vi "route.vi"() -> ()   [LabVIEW 2014]
uses:
  <vilib>/Utility/sysdir.llb/System Directory Type.ctl
  <vilib>/Utility/config.llb/Read Key (Path).vi
  subVI/departure.vi
  subVI/Destination.vi
  <vilib>/Utility/file.llb/Write To Spreadsheet File (string).vi
  <vilib>/Utility/config.llb/Write Key (Path).vi
  <vilib>/httpClient/LabVIEWHTTPClient.lvlib
  <vilib>/Utility/config.llb/NI_LVConfig.lvlib
panel:
  out "fms":string
  in  "날시":bool
  out "FUEL/연료":i32
  out "time/시간":dbl
  in  "도움말":bool
  in  "피드백":bool
  in  "저장 경로":path
  out "Distance":string="0"
  in  "찾기":bool
  in  "?":bool
  in  "?":bool
  out "x fmc 플랜":string
  out "FMS 플랜":string
  in  "Destination":string
  in  "departure":string
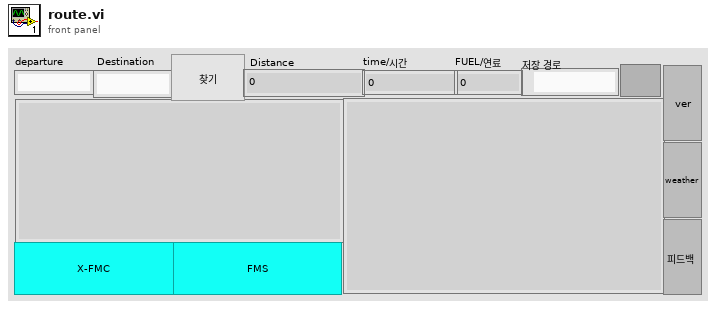
[diagram p1: front panel]
types:
  T1 = enum16{"open", "replace", "create", "open or create", "replace or create", "replace or create with confirmation"}
  T2 = typedef "System Directory Type.ctl" = i32
  T3 = typedef "NI_LVConfig.lvlib/Config Data RefNum.ctl" = refnum<k1>
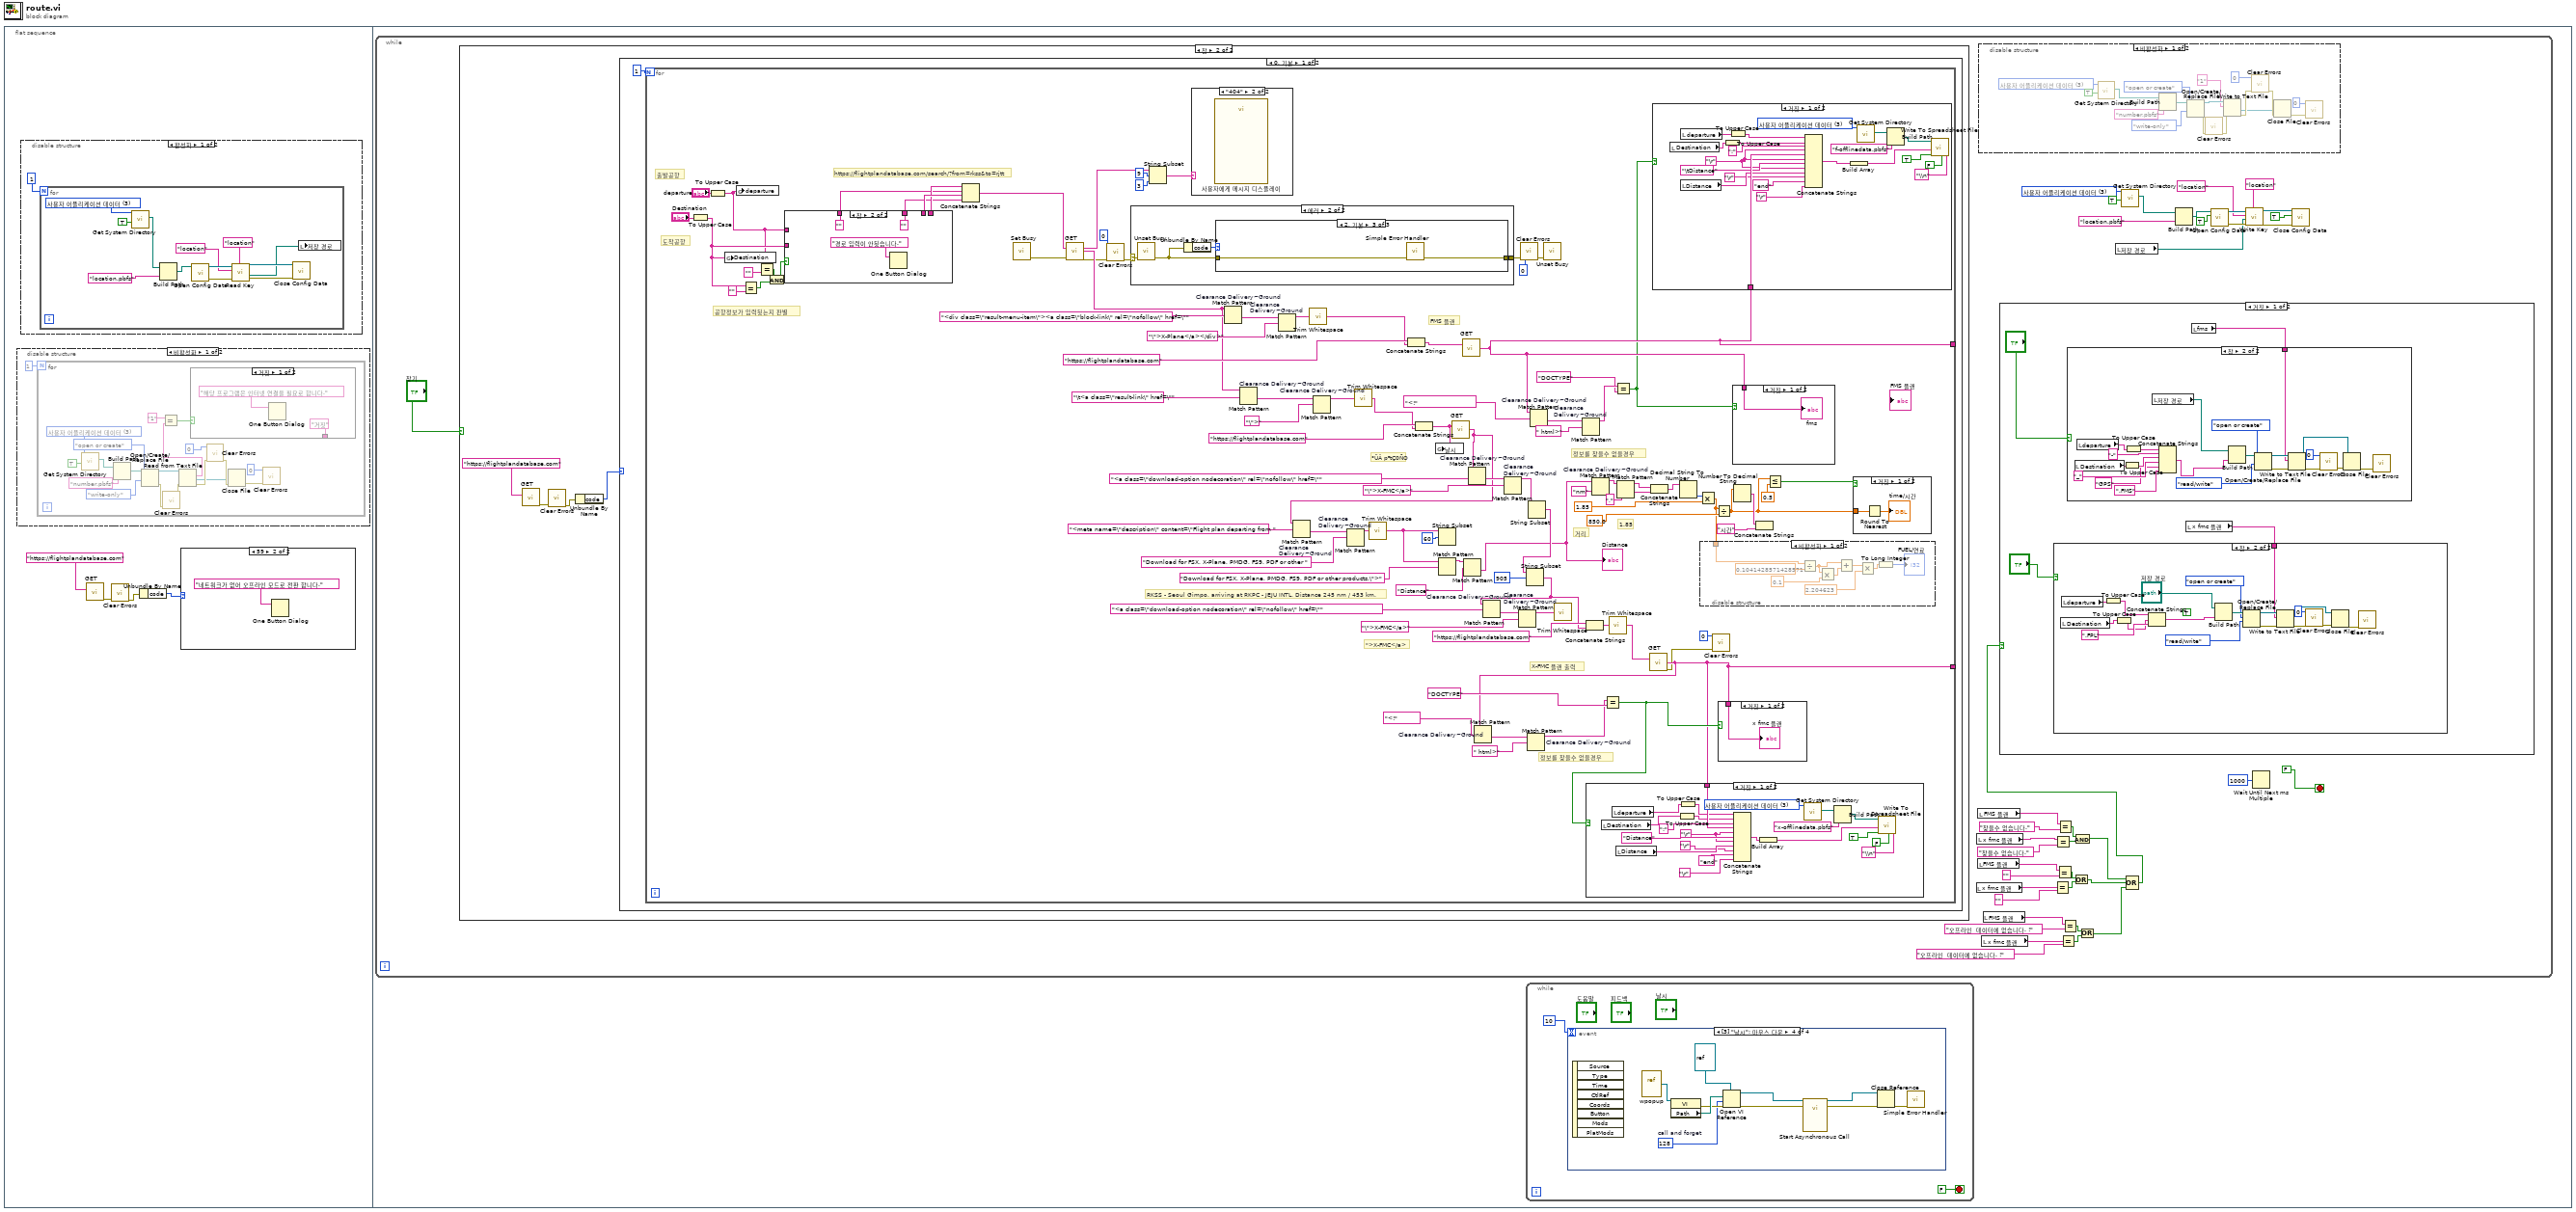
[diagram p0: block diagram]
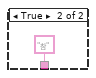
[diagram p3: hidden frame]
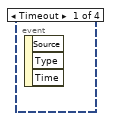
[diagram p6: hidden frame]
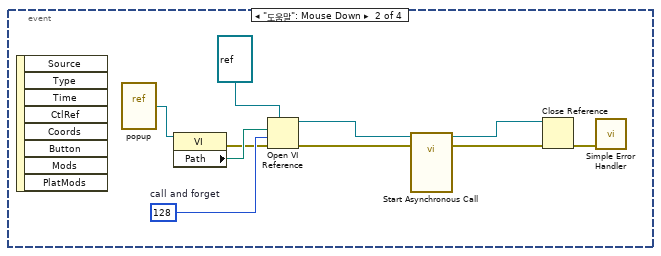
[diagram p7: hidden frame]
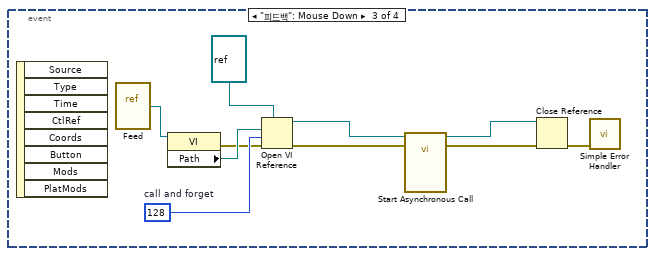
[diagram p8: hidden frame]
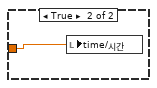
[diagram p13: hidden frame]
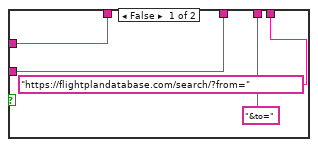
[diagram p14: hidden frame]
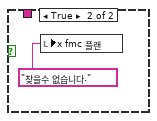
[diagram p15: hidden frame]
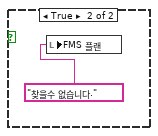
[diagram p16: hidden frame]
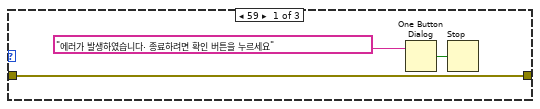
[diagram p19: hidden frame]
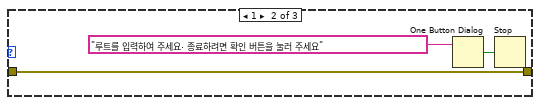
[diagram p20: hidden frame]
diagram:
  n1 = flat-sequence {
    frame #0 {
      n2 = disable-structure shown="비활성화" {
        frame Disabled {
          n3 = for {
            N: 1 -> [_]
            w12 = T2 3 items=["사용자 홈"=0, "사용자 데스크탑"=1, "사용자 문서"=2, "사용자 어플리케이션 데이터"=3, "사용자 환경"=4, "사용자 임시"=5, "퍼블릭 문서"=6, "퍼블릭 어플리케이션 데이터"=7, "퍼블릭 환경"=8, "퍼블릭 캐시"=13, "시스템 코어 라이브러리"=9, "시스템 설치된 라이브러리"=10, "어플리케이션 파일"=11, "부팅 볼륨 루트"=12] ("system directory type")
            n4 = call <vilib>:"Get System Directory.vi"("create directory if not found? (F)"=TRUE, "system directory type"=w12) -> ("system directory"=w13:path)  [unwired: 9 in]
            n5 = Build Path(base path=w13, name or relative path="number.pbfs" ("이름 또는 상대 경로")) -> (appended path=w18:path)
            n6 = Open/Create/Replace File(file path (use dialog)=w18, operation (0:open)=T1."open or create" ("동작(0:open)"), access (0:read/write)=enum16{"read/write", "read-only", "write-only"}."write-only" ("접근(0:읽기/쓰기)")) -> (refnum out=w21:refnum<file>, error out=w10:errorcluster)  [unwired: 3 in, 1 out]
            n7 = call <vilib>:"Clear Errors.vi"("error in (no error)"=w10) -> ("error out"=w9:errorcluster)  [unwired: 5 in, 1 out]
            n8 = Read from Text File(file (use dialog)=w21, error in=w9) -> (refnum out=w22:refnum<file>, text=w7:string, error out=w23:errorcluster)  [unwired: 2 in, 1 out]
            n9 = Equal?(x="1" ("y"), y=w7) -> (x = y?=w17:bool)
            n10 = case shown="거짓" w17 {
              tunnel: ["거짓" "참"] -> _
              frame False {
                n11 = One Button Dialog(message="해당 프로그램은 인터넷 연결을 필요로 합니다." ("메시지")) -> ()  [unwired: 1 in, 1 out]
              }
              frame True {
              }
            }
            n12 = call <vilib>:"Clear Errors.vi"("error in (no error)"=w23, "specific error code to clear (0: all)"=0) -> ("error out"=w24:errorcluster)  [unwired: 4 in, 1 out]
            n13 = Close File(refnum=w22, error in=w24) -> (error out=w15:errorcluster)  [unwired: 1 out]
            n14 = call <vilib>:"Clear Errors.vi"("error in (no error)"=w15, "specific error code to clear (0: all)"=0) -> ()  [unwired: 4 in, 2 out]
          }
        }
        frame Enabled {
        }
      }
      n15 = disable-structure shown="활성화" {
        frame Enabled {
          n16 = for {
            N: 1 -> [_]
            w40 = T2 3 items=["사용자 홈"=0, "사용자 데스크탑"=1, "사용자 문서"=2, "사용자 어플리케이션 데이터"=3, "사용자 환경"=4, "사용자 임시"=5, "퍼블릭 문서"=6, "퍼블릭 어플리케이션 데이터"=7, "퍼블릭 환경"=8, "퍼블릭 캐시"=13, "시스템 코어 라이브러리"=9, "시스템 설치된 라이브러리"=10, "어플리케이션 파일"=11, "부팅 볼륨 루트"=12] ("system directory type")
            n17 = call <vilib>:"Get System Directory.vi"("create directory if not found? (F)"=TRUE, "system directory type"=w40) -> ("system directory"=w38:path)  [unwired: 9 in]
            n18 = Build Path(base path=w38, name or relative path="location.pbfs" ("문자열")) -> (appended path=w37:path)
            n19 = call <vilib>:"Open Config Data.vi"("configuration file path"=w37) -> ("error out"=w34:errorcluster, "refnum"=w33:T3)  [unwired: 8 in, 1 out]
            n20 = call-poly <vilib>:"Read Key.vi"("section"="location", "error in (no error)"=w34, "key"="location", "refnum"=w33) -> ("error out"=w35:errorcluster, "value"=w30:path, "refnum out"=w36:T3)  [unwired: 4 in, 1 out]
            n21 = call <vilib>:"Close Config Data.vi"("error in (no error)"=w35, "refnum"=w36) -> ()  [unwired: 8 in, 2 out]
            n22 = local write "저장 경로"(w30) -> ()
          }
        }
        frame Disabled {
        }
      }
      n23 = call <vilib>:"GET.vi"("url"="https://flightplandatabase.com") -> ("error out"=w4:errorcluster)  [unwired: 11 in, 3 out]
      n24 = call <vilib>:"Clear Errors.vi"("error in (no error)"=w4) -> ("error out"=w2:errorcluster)  [unwired: 5 in, 1 out]
      n25 = Unbundle By Name(w2) -> ("code"=w1:i32)
      n26 = case shown="59" w1 {
        frame 0, Default {
        }
        frame 59 {
          n27 = One Button Dialog(message="네트워크가 없어 오프라인 모드로 전환 합니다." ("메시지")) -> ()  [unwired: 1 in, 1 out]
        }
      }
    }
    frame #1 {
      n28 = while {
        stop <- FALSE stop-if-true
        w94 = T2 3 items=["사용자 홈"=0, "사용자 데스크탑"=1, "사용자 문서"=2, "사용자 어플리케이션 데이터"=3, "사용자 환경"=4, "사용자 임시"=5, "퍼블릭 문서"=6, "퍼블릭 어플리케이션 데이터"=7, "퍼블릭 환경"=8, "퍼블릭 캐시"=13, "시스템 코어 라이브러리"=9, "시스템 설치된 라이브러리"=10, "어플리케이션 파일"=11, "부팅 볼륨 루트"=12] ("system directory type")
        n29 = case shown="참" "찾기" {
          frame False {
          }
          frame True {
            n30 = call <vilib>:"GET.vi"("url"="https://flightplandatabase.com") -> ("error out"=w116:errorcluster)  [unwired: 11 in, 3 out]
            n31 = call <vilib>:"Clear Errors.vi"("error in (no error)"=w116) -> ("error out"=w114:errorcluster)  [unwired: 5 in, 1 out]
            n32 = Unbundle By Name(w114) -> ("code"=w113:i32)
            n33 = case shown="0, 기본" w113 {
              frame 0, Default {
                n34 = for {
                  N: 1 -> [_]
                  tunnel: [w126] -> _
                  tunnel: [w132] -> _
                  # "°ÜÂ p³tÇ0ÑO"
                  # "1.85"
                  # "RKSS - Seoul Gimpo, arriving at RKPC - JEJU INTL. Distance 245 nm / 453 km."
                  # "\">X-FMC</a>"
                  # "https://flightplandatabase.com/search/?from=rkss&to=rjtt"
                  # "FMS 플랜"
                  # "거리"
                  # "X-FMC 플랜 출력"
                  # "정보를 찾을수 없을경우"
                  # "정보를 찾을수 없을경우"
                  # "공항정보가 입력됫는지 판별"
                  # "도착공항"
                  # "출발공항"
                  n35 = To Upper Case(1:"Destination") -> (0:w120:string)
                  n36 = To Upper Case(1:"departure") -> (0:w119:string)
                  n37 = global write "Destination.vi" "Destination"(w120) -> ()
                  n38 = global write "departure.vi" "departure"(w119) -> ()
                  n39 = Equal?(x=w120, y="") -> (x = y?=w158:bool)
                  n40 = Equal?(x=w119, y="") -> (x = y?=w157:bool)
                  n41 = And(x=w157, y=w158) -> (x .and. y?=w159:bool)
                  n42 = case shown="참" w159 {
                    tunnel: ["&to=" ("문자열") _] -> w149
                    tunnel: ["https://flightplandatabase.com/search/?from=" ("문자열") _] -> w148
                    tunnel: w120 -> [w269 _]
                    tunnel: [w269 "" ("Destination")] -> w147
                    tunnel: [w268 "" ("departure")] -> w146
                    tunnel: w119 -> [w268 _]
                    frame False {
                    }
                    frame True {
                      n43 = One Button Dialog(message="경로 입력이 안됫습니다." ("메시지")) -> ()  [unwired: 1 in, 1 out]
                    }
                  }
                  n44 = Concatenate Strings(w148, w146, w149, w147) -> (w130:string)
                  n45 = call <vilib>:"Set Busy.vi"() -> ("error out"=w209:errorcluster)  [unwired: 10 in, 1 out]
                  n46 = call <vilib>:"GET.vi"("url"=w130, "error in (no error)"=w209) -> ("headers"=w213:string, "body"=w183:string, "error out"=w168:errorcluster)  [unwired: 10 in, 1 out]
                  n47 = call <vilib>:"Clear Errors.vi"("error in (no error)"=w168, "specific error code to clear (0: all)"=0) -> ("error out"=w169:errorcluster)  [unwired: 4 in, 1 out]
                  n48 = case shown="에러" w169 {
                    selector: w169 -> [w279 w282]
                    tunnel: [w279 w280] -> w165
                    frame No Error {
                    }
                    frame Error {
                      n49 = call <vilib>:"Unset Busy.vi"("error in (no error)"=w282) -> ("error out"=w281:errorcluster)  [unwired: 10 in]
                      n50 = Unbundle By Name(w281) -> ("code"=w283:i32)
                      n51 = case shown="2, 기본" w283 {
                        tunnel: w281 -> [w284 w289 w291]
                        tunnel: [w284 w289 w290] -> w280
                        frame 59 {
                          n52 = One Button Dialog(message="에러가 발생하였습니다. 종료하려면 확인 버튼을 누르세요" ("메시지")) -> (true=w285:bool)  [unwired: 1 in]
                          n53 = Stop(stop? (T)=w285) -> ()
                        }
                        frame 1 {
                          n54 = One Button Dialog(message="루트를 입력하여 주세요. 종료하려면 확인 버튼을 눌러 주세요" ("메시지")) -> (true=w287:bool)  [unwired: 1 in]
                          n55 = Stop(stop? (T)=w287) -> ()
                        }
                        frame 2, Default {
                          n56 = call <vilib>:"Simple Error Handler.vi"("error in (no error)"=w291) -> ("error out"=w290:errorcluster)  [unwired: 4 in, 4 out]
                        }
                      }
                    }
                  }
                  n57 = String Subset(string=w213, offset (0)=9 ("오프셋(0)"), length (rest)=3 ("길이(나머지)")) -> (substring=w210:string)
                  n58 = case shown="\"404\"" w210 {
                    frame "거짓", Default {
                    }
                    frame "404" {
                      n59 = call "사용자에게 메시지 디스플레이"() -> ()  [unwired: 10 in, 2 out]
                    }
                  }
                  n60 = Match Pattern "Clearance Delivery~Ground"(string=w183, regular expression="<div class=\"result-menu-item\"><a class=\"block-link\" rel=\"nofollow\" href=\"" ("정규식")) -> (after substring=w207:string)  [unwired: 1 in, 3 out]
                  n61 = Match Pattern "Clearance Delivery~Ground"(string=w183, regular expression="\t<a class=\"result-link\" href=\"" ("정규식")) -> (after substring=w201:string)  [unwired: 1 in, 3 out]
                  n62 = Match Pattern "Clearance Delivery~Ground"(string=w207, regular expression="\">X-Plane</a></div>" ("정규식")) -> (before substring=w205:string)  [unwired: 1 in, 3 out]
                  n63 = call <vilib>:"Trim Whitespace.vi"("string"=w205) -> ("trimmed string"=w202:string)  [unwired: 1 in]
                  n64 = Match Pattern "Clearance Delivery~Ground"(string=w201, regular expression="\">" ("정규식")) -> (before substring=w198:string)  [unwired: 1 in, 3 out]
                  n65 = call <vilib>:"Trim Whitespace.vi"("string"=w198) -> ("trimmed string"=w196:string)  [unwired: 1 in]
                  n66 = Concatenate Strings("https://flightplandatabase.com" ("url"), w202) -> (w203:string)
                  n67 = Concatenate Strings("https://flightplandatabase.com" ("url"), w196) -> (w128:string)
                  n68 = global write "날시.vi" "날시"(w128) -> ()
                  n69 = call <vilib>:"GET.vi"("url"=w128) -> ("body"=w129:string)  [unwired: 11 in, 3 out]
                  n70 = Match Pattern "Clearance Delivery~Ground"(string=w129, regular expression="<meta name=\"description\" content=\"Flight plan departing from " ("정규식")) -> (after substring=w184:string)  [unwired: 1 in, 3 out]
                  n71 = Match Pattern "Clearance Delivery~Ground"(string=w184, regular expression="Download for FSX, X-Plane, PMDG, FS9, PDF or other " ("정규식")) -> (before substring=w186:string)  [unwired: 1 in, 3 out]
                  n72 = call <vilib>:"Trim Whitespace.vi"("string"=w186) -> ("trimmed string"=w154:string)  [unwired: 1 in]
                  n73 = String Subset(string=w154, offset (0)=60 ("오프셋(0)")) -> ()  [unwired: 1 in, 1 out]
                  n74 = Match Pattern(string=w154, regular expression="Download for FSX, X-Plane, PMDG, FS9, PDF or other products.\">" ("정규식")) -> (before substring=w152:string)  [unwired: 1 in, 3 out]
                  n75 = call <vilib>:"GET.vi"("url"=w203) -> ("body"=w132:string)  [unwired: 11 in, 3 out]
                  n76 = Match Pattern(string=w152, regular expression="Distance" ("정규식")) -> (after substring=w150:string)  [unwired: 1 in, 3 out]
                  "Distance" <- w150
                  n77 = Match Pattern "Clearance Delivery~Ground"(string=w129, regular expression="<a class=\"download-option nodecoration\" rel=\"nofollow\" href=\"" ("정규식")) -> (after substring=w193:string)  [unwired: 1 in, 3 out]
                  n78 = Match Pattern "Clearance Delivery~Ground"(string=w193, regular expression="\">X-FMC</a>" ("정규식")) -> (before substring=w192:string)  [unwired: 1 in, 3 out]
                  n79 = call <vilib>:"Clear Errors.vi"("error in (no error)"=w165, "specific error code to clear (0: all)"=0) -> ("error out"=w166:errorcluster)  [unwired: 4 in, 1 out]
                  n80 = String Subset(string=w192) -> (substring=w155:string)  [unwired: 2 in]
                  n81 = String Subset(string=w155, offset (0)=905 ("오프셋(0)")) -> (substring=w122:string)  [unwired: 1 in]
                  n82 = Match Pattern "Clearance Delivery~Ground"(string=w122, regular expression="<a class=\"download-option nodecoration\" rel=\"nofollow\" href=\"" ("정규식")) -> (after substring=w189:string)  [unwired: 1 in, 3 out]
                  n83 = Match Pattern "Clearance Delivery~Ground"(string=w189, regular expression="\">X-FMC</a>" ("정규식")) -> (before substring=w123:string)  [unwired: 1 in, 3 out]
                  n84 = Match Pattern "Clearance Delivery~Ground"(string=w132, regular expression="<!" ("문자열")) -> (after substring=w179:string)  [unwired: 1 in, 3 out]
                  n85 = call <vilib>:"Unset Busy.vi"("error in (no error)"=w166) -> ()  [unwired: 10 in, 1 out]
                  n86 = call <vilib>:"Trim Whitespace.vi"("string"=w123) -> ()  [unwired: 1 in, 1 out]
                  n87 = Match Pattern "Clearance Delivery~Ground"(string=w179, regular expression=" html>" ("정규식")) -> (before substring=w178:string)  [unwired: 1 in, 3 out]
                  n88 = Concatenate Strings("https://flightplandatabase.com" ("url"), w122) -> (w187:string)
                  n89 = Match Pattern "Clearance Delivery~Ground"(string=w150, regular expression="nm" ("정규식")) -> (before substring=w142:string)  [unwired: 1 in, 3 out]
                  n90 = call <vilib>:"Trim Whitespace.vi"("string"=w187) -> ("trimmed string"=w127:string)  [unwired: 1 in]
                  n91 = Equal?(x=w178, y="DOCTYPE") -> (x = y?=w131:bool)
                  n92 = Match Pattern(string=w142, regular expression="," ("정규식")) -> (before substring=w139:string, after substring=w138:string)  [unwired: 1 in, 2 out]
                  n93 = call <vilib>:"GET.vi"("url"=w127) -> ("body"=w126:string, "error out"=w125:errorcluster)  [unwired: 11 in, 2 out]
                  n94 = Match Pattern "Clearance Delivery~Ground"(string=w126, regular expression="<!" ("문자열")) -> (after substring=w176:string)  [unwired: 1 in, 3 out]
                  n95 = Match Pattern "Clearance Delivery~Ground"(string=w176, regular expression=" html>" ("정규식")) -> (before substring=w173:string)  [unwired: 1 in, 3 out]
                  n96 = Equal?(x=w173, y="DOCTYPE") -> (x = y?=w133:bool)
                  n97 = case shown="거짓" w133 {
                    tunnel: w126 -> [w254 _]
                    frame False {
                      w248 = "\r"
                      w257 = T2 3 items=["사용자 홈"=0, "사용자 데스크탑"=1, "사용자 문서"=2, "사용자 어플리케이션 데이터"=3, "사용자 환경"=4, "사용자 임시"=5, "퍼블릭 문서"=6, "퍼블릭 어플리케이션 데이터"=7, "퍼블릭 환경"=8, "퍼블릭 캐시"=13, "시스템 코어 라이브러리"=9, "시스템 설치된 라이브러리"=10, "어플리케이션 파일"=11, "부팅 볼륨 루트"=12] ("system directory type")
                      n98 = local read "Destination"() -> (w250:string)
                      n99 = local read "departure"() -> (w253:string)
                      n100 = local read "Distance"() -> (w247:string)
                      n101 = To Upper Case(1:w250) -> (0:w251:string)
                      n102 = To Upper Case(1:w253) -> (0:w252:string)
                      n103 = Concatenate Strings(w252, w251, ":", w254, w248, "Distance" ("문자열"), w248, w247, "\r", "end", "\r") -> (w255:string)
                      n104 = Build Array(w255) -> (w259:string[])
                      n105 = call <vilib>:"Get System Directory.vi"("system directory type"=w257) -> ("system directory"=w261:path)  [unwired: 10 in]
                      n106 = Build Path(base path=w261, name or relative path="x-offlinedata.pbfs" ("이름 또는 상대 경로")) -> (appended path=w260:path)
                      n107 = call-poly <vilib>:"Write To Spreadsheet File.vi"("delimiter (\\t)"="\\n" ("delimiter (\\t)"), "transpose? (no:F)"=FALSE, "append to file? (new file:F)"=TRUE, "1D data"=w259, "file path (dialog if empty)"=w260) -> ()  [unwired: 3 in, 1 out]
                    }
                    frame True {
                    }
                  }
                  n108 = Concatenate Strings(w139, w138) -> (w141:string)
                  n109 = case shown="거짓" w131 {
                    tunnel: w132 -> [w229 _]
                    frame False {
                      w227 = "\r"
                      w236 = T2 3 items=["사용자 홈"=0, "사용자 데스크탑"=1, "사용자 문서"=2, "사용자 어플리케이션 데이터"=3, "사용자 환경"=4, "사용자 임시"=5, "퍼블릭 문서"=6, "퍼블릭 어플리케이션 데이터"=7, "퍼블릭 환경"=8, "퍼블릭 캐시"=13, "시스템 코어 라이브러리"=9, "시스템 설치된 라이브러리"=10, "어플리케이션 파일"=11, "부팅 볼륨 루트"=12] ("system directory type")
                      n110 = local read "Destination"() -> (w230:string)
                      n111 = local read "Distance"() -> (w226:string)
                      n112 = local read "departure"() -> (w232:string)
                      n113 = To Upper Case(1:w230) -> (0:w231:string)
                      n114 = To Upper Case(1:w232) -> (0:w233:string)
                      n115 = Concatenate Strings(w233, w231, ":", w227, w229, w227, "\tDistance", w227, w226, "\r", "end", "\r") -> (w234:string)
                      n116 = Build Array(w234) -> (w238:string[])
                      n117 = call <vilib>:"Get System Directory.vi"("system directory type"=w236) -> ("system directory"=w240:path)  [unwired: 10 in]
                      n118 = Build Path(base path=w240, name or relative path="f-offlinedata.pbfs" ("이름 또는 상대 경로")) -> (appended path=w239:path)
                      n119 = call-poly <vilib>:"Write To Spreadsheet File.vi"("delimiter (\\t)"="\\n" ("delimiter (\\t)"), "transpose? (no:F)"=FALSE, "append to file? (new file:F)"=TRUE, "1D data"=w238, "file path (dialog if empty)"=w239) -> ()  [unwired: 3 in, 1 out]
                    }
                    frame True {
                    }
                  }
                  n120 = Decimal String To Number(string=w141) -> (number=w143:i32)  [unwired: 2 in, 1 out]
                  n121 = Multiply(x=w143, y=1.85) -> (x*y=w134:dbl)
                  n122 = disable-structure shown="비활성화" {
                    disable-tunnel: w134 -> [w219 _]
                    frame Disabled {
                      n123 = Divide(x=w219, y=0.1041428571428571) -> (x/y=w220:dbl)
                      n124 = Multiply(x=w220, y=0.1) -> (x*y=w218:dbl)
                      n125 = Add(x=w220, y=w218) -> (x+y=w217:dbl)
                      n126 = Multiply(x=w217, y=2.204623) -> (x*y=w214:dbl)
                      n127 = To Long Integer(number=w214) -> (32bit integer=→"FUEL/연료":i32)
                    }
                    frame Enabled {
                    }
                  }
                  n128 = call <vilib>:"Clear Errors.vi"("error in (no error)"=w125, "specific error code to clear (0: all)"=0) -> ()  [unwired: 4 in, 2 out]
                  n129 = Divide(x=w134, y=850.0) -> (x/y=w135:dbl)
                  n130 = case shown="거짓" w133 {
                    tunnel: w126 -> [w275 _]
                    frame False {
                      "x fmc 플랜" <- w275
                    }
                    frame True {
                      n131 = local write "x fmc 플랜"("찾을수 없습니다.") -> ()
                    }
                  }
                  n132 = case shown="거짓" w131 {
                    tunnel: w132 -> [w277 _]
                    frame False {
                      "fms" <- w277
                    }
                    frame True {
                      n133 = local write "FMS 플랜"("찾을수 없습니다.") -> ()
                    }
                  }
                  n134 = Number To Decimal String(number=w135) -> (decimal integer string=w160:string)  [unwired: 1 in]
                  n135 = Concatenate Strings(w160, "시간") -> ()  [unwired: 1 out]
                  n136 = Less Or Equal?(x=w135, y=0.5) -> (x <= y?=w137:bool)
                  n137 = case shown="거짓" w137 {
                    tunnel: w135 -> [w266 w267]
                    frame False {
                      n138 = Round To Nearest(number=w266) -> (nearest integer value=→"time/시간":dbl)
                    }
                    frame True {
                      n139 = local write "time/시간"(w267) -> ()
                    }
                  }
                }
              }
              frame 59 {
                n140 = while {
                  stop <- FALSE stop-if-true
                  w292 = "Distance" ("정규식")
                  w329 = T2 1 items=["사용자 홈"=0, "사용자 데스크탑"=1, "사용자 문서"=2, "사용자 어플리케이션 데이터"=3, "사용자 환경"=4, "사용자 임시"=5, "퍼블릭 문서"=6, "퍼블릭 어플리케이션 데이터"=7, "퍼블릭 환경"=8, "퍼블릭 캐시"=13, "시스템 코어 라이브러리"=9, "시스템 설치된 라이브러리"=10, "어플리케이션 파일"=11, "부팅 볼륨 루트"=12] ("system directory type")
                  w343 = T2 1 items=["사용자 홈"=0, "사용자 데스크탑"=1, "사용자 문서"=2, "사용자 어플리케이션 데이터"=3, "사용자 환경"=4, "사용자 임시"=5, "퍼블릭 문서"=6, "퍼블릭 어플리케이션 데이터"=7, "퍼블릭 환경"=8, "퍼블릭 캐시"=13, "시스템 코어 라이브러리"=9, "시스템 설치된 라이브러리"=10, "어플리케이션 파일"=11, "부팅 볼륨 루트"=12] ("system directory type")
                  n141 = local read "Destination"() -> (w323:string)
                  n142 = local read "departure"() -> (w325:string)
                  n143 = call <vilib>:"Get System Directory.vi"("system directory type"=w329) -> ("system directory"=w328:path)  [unwired: 10 in]
                  n144 = call <vilib>:"Get System Directory.vi"("system directory type"=w343) -> ("system directory"=w344:path)  [unwired: 10 in]
                  n145 = To Upper Case(1:w323) -> (0:w322:string)
                  n146 = Build Path(base path=w328, name or relative path="f-offlinedata.pbfs" ("이름 또는 상대 경로")) -> (appended path=w331:path)
                  n147 = To Upper Case(1:w325) -> (0:w324:string)
                  n148 = Build Path(base path=w344, name or relative path="x-offlinedata.pbfs" ("이름 또는 상대 경로")) -> (appended path=w341:path)
                  n149 = Concatenate Strings(w324, w322, ":") -> (w319:string)
                  n150 = Read from Text File(file (use dialog)=w331) -> (refnum out=w332:refnum<file>, text=w317:string, error out=w333:errorcluster)  [unwired: 3 in, 1 out]
                  n151 = Read from Text File(file (use dialog)=w341) -> (refnum out=w340:refnum<file>, text=w293:string, error out=w339:errorcluster)  [unwired: 3 in, 1 out]
                  n152 = Close File(refnum=w332, error in=w333) -> ()  [unwired: 2 out]
                  n153 = Close File(refnum=w340, error in=w339) -> ()  [unwired: 2 out]
                  n154 = Match Pattern(string=w293, regular expression=w319) -> (after substring=w321:string)  [unwired: 1 in, 3 out]
                  n155 = Match Pattern(string=w317, regular expression=w319) -> (after substring=w326:string)  [unwired: 1 in, 3 out]
                  n156 = Match Pattern(string=w326, regular expression="Distance") -> (before substring=w327:string)  [unwired: 1 in, 3 out]
                  n157 = Match Pattern(string=w321, regular expression=w292) -> (before substring=w320:string)  [unwired: 1 in, 3 out]
                  n158 = Match Pattern(string=w293, regular expression=w292) -> (after substring=w316:string)  [unwired: 1 in, 3 out]
                  n159 = Match Pattern(string=w316, regular expression="end" ("정규식")) -> (before substring=w306:string)  [unwired: 1 in, 3 out]
                  n160 = Equal?(x=w320, y="") -> (x = y?=w338:bool)
                  n161 = call <vilib>:"Trim Whitespace.vi"("string"=w306) -> ("trimmed string"=w312:string)  [unwired: 1 in]
                  n162 = Match Pattern "time/fuel"(string=w312, regular expression="nm" ("정규식")) -> (before substring=w308:string)  [unwired: 1 in, 3 out]
                  n163 = Match Pattern(string=w308, regular expression="," ("정규식")) -> (before substring=w310:string, after substring=w311:string)  [unwired: 1 in, 2 out]
                  n164 = Concatenate Strings(w310, w311) -> (w309:string)
                  n165 = Decimal String To Number(string=w309) -> (number=w297:i32)  [unwired: 2 in, 1 out]
                  n166 = Multiply(x=w297, y=1.85) -> (x*y=w296:dbl)
                  n167 = Divide(x=w296, y=850.0) -> (x/y=w294:dbl)
                  n168 = Equal?(x=w327, y="") -> (x = y?=w335:bool)
                  n169 = case shown="거짓" w335 {
                    tunnel: w327 -> [w346 _]
                    frame False {
                      n170 = local write "FMS 플랜"(w346) -> ()
                    }
                    frame True {
                      n171 = local write "x fmc 플랜"("오프라인  데이터에 없습니다. !" ("메시지")) -> ()
                    }
                  }
                  n172 = Divide(x=w296, y=0.1041428571428571) -> (x/y=w300:dbl)
                  n173 = Multiply(x=w300, y=0.1) -> (x*y=w301:dbl)
                  n174 = Add(x=w300, y=w301) -> (x+y=w302:dbl)
                  n175 = Multiply(x=w302, y=2.204623) -> (x*y=w304:dbl)
                  n176 = To Long Integer(number=w304) -> (32bit integer=w295:i32)
                  n177 = case shown="거짓" w338 {
                    tunnel: w320 -> [w353 _]
                    tunnel: w295 -> [w348 _]
                    tunnel: w294 -> [w349 _]
                    tunnel: w294 -> [w350 _]
                    frame False {
                      n178 = Less Or Equal?(x=w350, y=0.5) -> (x <= y?=w352:bool)
                      n179 = local write "x fmc 플랜"(w353) -> ()
                      n180 = case shown="거짓" w352 {
                        tunnel: w349 -> [w354 w356]
                        frame False {
                          n181 = Round To Nearest(number=w354) -> (nearest integer value=w355:dbl)
                          n182 = local write "time/시간"(w355) -> ()
                        }
                        frame True {
                          n183 = local write "time/시간"(w356) -> ()
                        }
                      }
                      n184 = local write "FUEL/연료"(w348) -> ()
                    }
                    frame True {
                      n185 = local write "x fmc 플랜"("오프라인  데이터에 없습니다. !" ("메시지")) -> ()
                    }
                  }
                }
              }
            }
          }
        }
        n186 = local read "x fmc 플랜"() -> (w101:string)
        n187 = local read "x fmc 플랜"() -> (w109:string)
        n188 = local read "FMS 플랜"() -> (w96:string)
        n189 = local read "FMS 플랜"() -> (w107:string)
        n190 = disable-structure shown="비활성화" {
          frame Disabled {
            w361 = T2 3 items=["사용자 홈"=0, "사용자 데스크탑"=1, "사용자 문서"=2, "사용자 어플리케이션 데이터"=3, "사용자 환경"=4, "사용자 임시"=5, "퍼블릭 문서"=6, "퍼블릭 어플리케이션 데이터"=7, "퍼블릭 환경"=8, "퍼블릭 캐시"=13, "시스템 코어 라이브러리"=9, "시스템 설치된 라이브러리"=10, "어플리케이션 파일"=11, "부팅 볼륨 루트"=12] ("system directory type")
            n191 = call <vilib>:"Get System Directory.vi"("create directory if not found? (F)"=TRUE, "system directory type"=w361) -> ("system directory"=w362:path)  [unwired: 9 in]
            n192 = Build Path(base path=w362, name or relative path="number.pbfs" ("이름 또는 상대 경로")) -> (appended path=w367:path)
            n193 = Open/Create/Replace File(file path (use dialog)=w367, operation (0:open)=T1."open or create" ("동작(0:open)"), access (0:read/write)=enum16{"read/write", "read-only", "write-only"}."write-only" ("접근(0:읽기/쓰기)")) -> (refnum out=w370:refnum<file>, error out=w359:errorcluster)  [unwired: 3 in, 1 out]
            n194 = call <vilib>:"Clear Errors.vi"("error in (no error)"=w359) -> ("error out"=w358:errorcluster)  [unwired: 5 in, 1 out]
            n195 = Write to Text File(file (use dialog)=w370, text="1" ("텍스트"), error in=w358) -> (refnum out=w371:refnum<file>, error out=w372:errorcluster)  [unwired: 1 in, 1 out]
            n196 = call <vilib>:"Clear Errors.vi"("error in (no error)"=w372, "specific error code to clear (0: all)"=0) -> ("error out"=w373:errorcluster)  [unwired: 4 in, 1 out]
            n197 = Close File(refnum=w371, error in=w373) -> (error out=w364:errorcluster)  [unwired: 1 out]
            n198 = call <vilib>:"Clear Errors.vi"("error in (no error)"=w364, "specific error code to clear (0: all)"=0) -> ()  [unwired: 4 in, 2 out]
          }
          frame Enabled {
          }
        }
        n199 = local read "x fmc 플랜"() -> (w78:string)
        n200 = local read "FMS 플랜"() -> (w74:string)
        n201 = Equal?(x=w101, y="") -> (x = y?=w103:bool)
        n202 = Equal?(x=w109, y="찾을수 없습니다.") -> (x = y?=w110:bool)
        n203 = Equal?(x=w96, y="") -> (x = y?=w102:bool)
        n204 = Equal?(x=w107, y="찾을수 없습니다.") -> (x = y?=w111:bool)
        n205 = Equal?(x=w78, y="오프라인  데이터에 없습니다. !") -> (x = y?=w76:bool)
        n206 = Equal?(x=w74, y="오프라인  데이터에 없습니다. !") -> (x = y?=w77:bool)
        n207 = Or(x=w102, y=w103) -> (x .or. y?=w91:bool)
        n208 = And(x=w111, y=w110) -> (x .and. y?=w98:bool)
        n209 = Or(x=w77, y=w76) -> (x .or. y?=w75:bool)
        n210 = local read "저장 경로"() -> (w82:path)
        n211 = call <vilib>:"Get System Directory.vi"("create directory if not found? (F)"=TRUE, "system directory type"=w94) -> ("system directory"=w92:path)  [unwired: 9 in]
        n212 = Compound Arithmetic op=OR(w98, w91, w75) -> (w97:bool)
        n213 = case shown="거짓" w97 {
          frame False {
            n214 = local read "x fmc 플랜"() -> (w375:string)
            n215 = case shown="참" "?" {
              tunnel: w375 -> [_ w401]
              frame False {
              }
              frame True {
                (unwired) TRUE ("create directory if not found? (F)")
                n216 = local read "Destination"() -> (w408:string)
                n217 = local read "departure"() -> (w409:string)
                n218 = To Upper Case(1:w409) -> (0:w400:string)
                n219 = To Upper Case(1:w408) -> (0:w407:string)
                n220 = Concatenate Strings(w400, w407, ".FPL" ("문자열")) -> (w412:string)
                n221 = Build Path(base path="저장 경로", name or relative path=w412) -> (appended path=w415:path)
                n222 = Open/Create/Replace File(file path (use dialog)=w415, operation (0:open)=T1."open or create" ("동작(0:open)"), access (0:read/write)=enum16{"read/write", "read-only", "write-only"}."read/write" ("접근(0:읽기/쓰기)")) -> (refnum out=w417:refnum<file>, error out=w416:errorcluster)  [unwired: 3 in, 1 out]
                n223 = Write to Text File(file (use dialog)=w417, text=w401, error in=w416) -> (refnum out=w404:refnum<file>, error out=w406:errorcluster)  [unwired: 1 in, 1 out]
                n224 = call <vilib>:"Clear Errors.vi"("error in (no error)"=w406, "specific error code to clear (0: all)"=0) -> ("error out"=w405:errorcluster)  [unwired: 4 in, 1 out]
                n225 = Close File(refnum=w404, error in=w405) -> (error out=w402:errorcluster)  [unwired: 1 out]
                n226 = call <vilib>:"Clear Errors.vi"("error in (no error)"=w402) -> ()  [unwired: 5 in, 2 out]
              }
            }
            n227 = local read "fms"() -> (w377:string)
            n228 = case shown="참" "?" {
              tunnel: w377 -> [_ w394]
              frame False {
              }
              frame True {
                n229 = local read "Destination"() -> (w391:string)
                n230 = local read "departure"() -> (w390:string)
                n231 = To Upper Case(1:w391) -> (0:w382:string)
                n232 = To Upper Case(1:w390) -> (0:w384:string)
                n233 = local read "저장 경로"() -> (w386:path)
                n234 = Concatenate Strings(w384, "-" ("문자열"), w382, "_" ("문자열"), "GPS" ("문자열"), ".FMS" ("문자열")) -> (w392:string)
                n235 = Build Path(base path=w386, name or relative path=w392) -> (appended path=w396:path)
                n236 = Open/Create/Replace File(file path (use dialog)=w396, operation (0:open)=T1."open or create" ("동작(0:open)"), access (0:read/write)=enum16{"read/write", "read-only", "write-only"}."read/write" ("접근(0:읽기/쓰기)")) -> (refnum out=w399:refnum<file>, error out=w398:errorcluster)  [unwired: 3 in, 1 out]
                n237 = Write to Text File(file (use dialog)=w399, text=w394, error in=w398) -> (refnum out=w397:refnum<file>, error out=w389:errorcluster)  [unwired: 1 in, 1 out]
                n238 = call <vilib>:"Clear Errors.vi"("error in (no error)"=w389, "specific error code to clear (0: all)"=0) -> ("error out"=w388:errorcluster)  [unwired: 4 in, 1 out]
                n239 = Close File(refnum=w397, error in=w388) -> (error out=w385:errorcluster)  [unwired: 1 out]
                n240 = call <vilib>:"Clear Errors.vi"("error in (no error)"=w385) -> ()  [unwired: 5 in, 2 out]
              }
            }
          }
          frame True {
          }
        }
        n241 = Build Path(base path=w92, name or relative path="location.pbfs" ("문자열")) -> (appended path=w90:path)
        n242 = call <vilib>:"Open Config Data.vi"("create file if necessary (T)"=TRUE, "configuration file path"=w90) -> ("error out"=w88:errorcluster, "refnum"=w87:T3)  [unwired: 7 in, 1 out]
        n243 = call-poly <vilib>:"Write Key.vi"("section"="location", "error in (no error)"=w88, "value"=w82, "key"="location", "refnum"=w87) -> ("error out"=w85:errorcluster, "refnum out"=w86:T3)  [unwired: 4 in, 1 out]
        n244 = Wait Until Next ms Multiple(millisecond multiple=u32 1000 ("ms 배수")) -> ()  [unwired: 1 out]
        n245 = call <vilib>:"Close Config Data.vi"("error in (no error)"=w85, "write file if changed (T)"=TRUE, "refnum"=w86) -> ()  [unwired: 7 in, 2 out]
      }
      n246 = while {
        stop <- FALSE stop-if-true
        n247 = event shown="[3] \"날시\": 마우스 다운" {
          selector: _ -> [_ _ _ _]
          dyn-events: _ -> [_ _ _ _]
          timeout: 10 -> [_ _ _ _]
          event Timeout {
            n248 = event-data() -> ()  [unwired: 1 in, 3 out]
          }
          event "도움말": Mouse Down {
            w53 = 128  # call and forget
            n249 = event-data() -> ()  [unwired: 1 in, 8 out]
            n250 = vi-ref "popup.vi"() -> (w46:refnum<vi>)
            n251 = property class="VI"(reference=w46) -> (error out=w47:errorcluster, "Path"=w48:path)  [unwired: 1 in, 1 out]
            n252 = Open VI Reference(type specifier VI Refnum (for type only)=refnum<vi> refnum, vi path=w48, options=w53, error in (no error)=w47) -> (vi reference=w45:refnum<vi>, error out=w51:errorcluster)  [unwired: 2 in]
            n253 = call-by-ref "Start Asynchronous Call"(reference=w45, error in=w51) -> (reference out=w44:refnum<vi>, error out=w50:errorcluster)  [unwired: 12 in]
            n254 = Close Reference(reference=w44, error in (no error)=w50) -> (error out=w49:errorcluster)
            n255 = call <vilib>:"Simple Error Handler.vi"("error in (no error)"=w49) -> ()  [unwired: 4 in, 5 out]
          }
          event "피드백": Mouse Down {
            w63 = 128  # call and forget
            n256 = event-data() -> ()  [unwired: 1 in, 8 out]
            n257 = vi-ref "Feed.vi"() -> (w56:refnum<vi>)
            n258 = property class="VI"(reference=w56) -> (error out=w57:errorcluster, "Path"=w58:path)  [unwired: 1 in, 1 out]
            n259 = Open VI Reference(type specifier VI Refnum (for type only)=refnum<vi> refnum, vi path=w58, options=w63, error in (no error)=w57) -> (vi reference=w55:refnum<vi>, error out=w61:errorcluster)  [unwired: 2 in]
            n260 = call-by-ref "Start Asynchronous Call"(reference=w55, error in=w61) -> (reference out=w54:refnum<vi>, error out=w60:errorcluster)  [unwired: 12 in]
            n261 = Close Reference(reference=w54, error in (no error)=w60) -> (error out=w59:errorcluster)
            n262 = call <vilib>:"Simple Error Handler.vi"("error in (no error)"=w59) -> ()  [unwired: 4 in, 5 out]
          }
          event "날시": Mouse Down {
            w64 = 128  # call and forget
            n263 = event-data() -> ()  [unwired: 1 in, 8 out]
            n264 = vi-ref "wpopup.vi"() -> (w67:refnum<vi>)
            n265 = property class="VI"(reference=w67) -> (error out=w68:errorcluster, "Path"=w69:path)  [unwired: 1 in, 1 out]
            n266 = Open VI Reference(type specifier VI Refnum (for type only)=refnum<vi> refnum, vi path=w69, options=w64, error in (no error)=w68) -> (vi reference=w66:refnum<vi>, error out=w72:errorcluster)  [unwired: 2 in]
            n267 = call-by-ref "Start Asynchronous Call"(reference=w66, error in=w72) -> (reference out=w65:refnum<vi>, error out=w71:errorcluster)  [unwired: 12 in]
            n268 = Close Reference(reference=w65, error in (no error)=w71) -> (error out=w70:errorcluster)
            n269 = call <vilib>:"Simple Error Handler.vi"("error in (no error)"=w70) -> ()  [unwired: 4 in, 5 out]
          }
        }
      }
    }
  }
